vi "CONV 2D Hexidecimal Array to String.vi"(0 "2-D Hexidecimal":u32[][](array[numeric]) format="%.0x", 1 "Delimiters (,;)":string=",;") -> (6 "String":string)   [LabVIEW 2012]
doc: "This routine converts a 2-D U32 Hexidecimal Array into a String list. There must be exactly 2 characters in the delimiters field. The first character is the Column Delimiter, and the second character is the Row Delimiter.\n\nExample:\n\n2-D String Input:\n\n1 2 3\n4 5 6\n\nDelimiters:\n,;\n\nString Output:\n\n1,2,3;4,5,6"
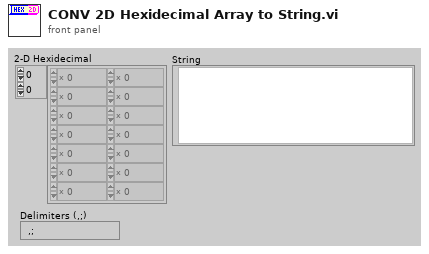
[diagram p1: front panel]
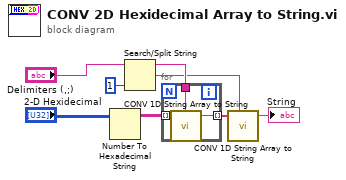
[diagram p0: block diagram]
diagram:
  n1 = Number To Hexadecimal String(2:"2-D Hexidecimal") -> (0:w2:string[][])  [unwired: 1 in]
  n2 = Search/Split String(string="Delimiters (,;)", offset (0)=1) -> (substring before match=w4:string, match + rest of string=w3:string)  [unwired: 1 in, 1 out]
  n3 = for {
    tunnel: w2 -> [w11] mode=indexing
    tunnel: [w10] -> w8 mode=indexing
    tunnel: w4 -> [w9]
    n4 = call "CONV 1D String Array to String.vi"("1-D String"=w11, "Delimiter (,)"=w9) -> ("String"=w10:string)  [unwired: 7 in]
  }
  n5 = call "CONV 1D String Array to String.vi"("1-D String"=w8, "Delimiter (,)"=w3) -> ("String"=→"String":string)  [unwired: 7 in]
